vi "Command (read) - MV.vi"(7 "timeout ms (100)":i32=100, 8 "error in (no error)":errorcluster, 10 "IP":string, 11 "connection ID in":refnum<k16>) -> (0 "error out":errorcluster, 2 "Model & Revision":string, 3 "connection ID out":refnum<k16>)   [LabVIEW 2016, in "SMD-7615.lvlib" / "eSCL.lvlib"]
doc: "MV - Model & Revision\nRequests the connected drive’s DSP firmware version, model number code, and sub-model number code (if applicable). Not all drive series utilize the sub-model number code. The response from the drive is a single string of characters with no breaks or delimiters. The sequence of characters is firmware revision (3 numbers and 1 letter), model number code (3 numbers), sub-model number code (1 letter)."
uses:
  eSCL.lvlib
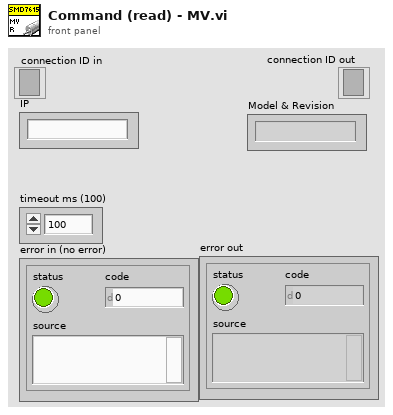
[diagram p1: front panel]
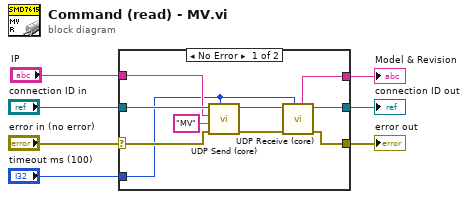
[diagram p0: block diagram]
diagram:
  n1 = case shown="No Error" "error in (no error)" {
    selector: "error in (no error)" -> [w13 w18]
    tunnel: "connection ID in" -> [w12 w19]
    tunnel: [w15 w19] -> w5
    tunnel: [w14 w18] -> w4
    tunnel: "IP" -> [w11 _]
    tunnel: "timeout ms (100)" -> [w9 _]
    tunnel: [w8 _] -> w1
    frame No Error {
      n2 = call "UDP Send (core).vi"("timeout ms (100)"=w9, "error in (no error)"=w13, "Data"="MV", "IP"=w11, "connection ID in"=w12) -> ("error out"=w17:errorcluster, "connection ID out"=w16:refnum<k16>)  [unwired: 5 in]
      n3 = call "UDP Receive (core).vi"("timeout ms (100)"=w9, "error in (no error)"=w17, "connection ID in"=w16) -> ("error out"=w14:errorcluster, "connection ID out"=w15:refnum<k16>, "Received String"=w8:string)  [unwired: 4 in, 2 out]
    }
    frame Error {
    }
  }
  "connection ID out" <- w5
  "error out" <- w4
  "Model & Revision" <- w1
